vi "ErrorLog_GetErrors.vi"(7 "Owner":string, 8 "error in (no error)":errorcluster, 11 "reference in":refnum<class "ErrorLog.lvclass">) -> (0 "error out":errorcluster, 1 "Errors since last call":string, 2 "New Errors":bool, 3 "reference out":refnum<class "ErrorLog.lvclass">, 4 "Errors since last clear":string, 5 "Uncleared Errors":bool)   [LabVIEW 2014, in "ErrorLog.lvclass"]
uses:
  ErrorLog.lvclass
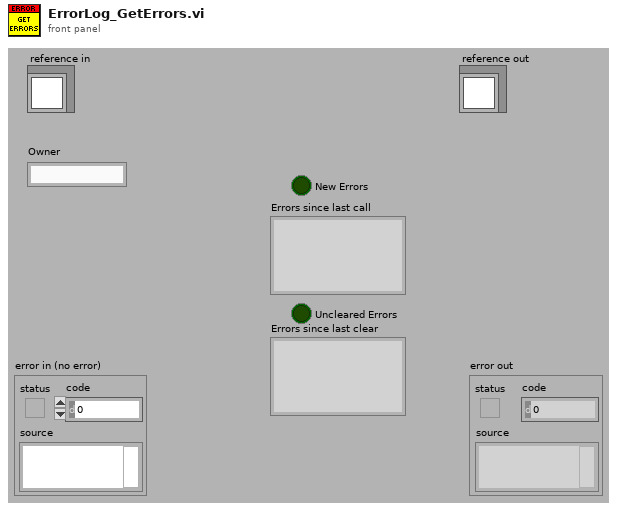
[diagram p1: front panel]
types:
  T1 = typedef "ErrorLog.lvclass/ObjectAttributes.ctl" = cluster{"ErrorFile":path, "Supress Consecutive Duplicates":bool, "Errors":string, "Quit":bool, "Errors since last call":string, "Last Recorded Error":string, "ErrorPath":path, "PossiblePaths":path[], "BaseFileName":string, "Max Log Files":i32, "ErrorFile Index":i32, "Max File Size":i64}
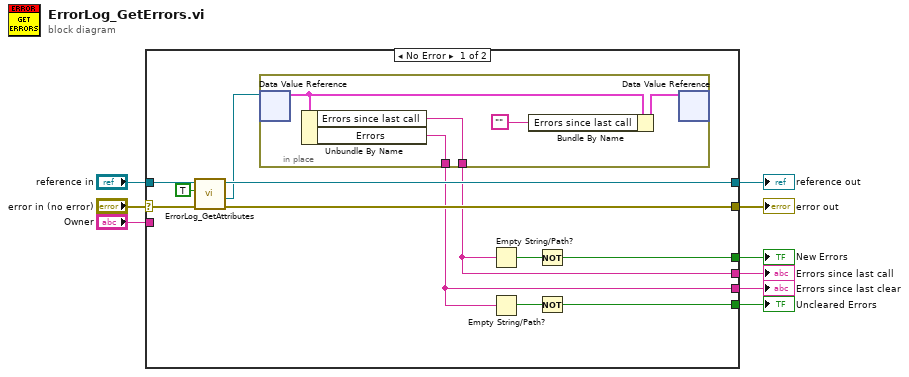
[diagram p0: block diagram]
diagram:
  n1 = case shown="No Error" "error in (no error)" {
    selector: "error in (no error)" -> [w21 w28]
    tunnel: [w19 w28] -> w8
    tunnel: [w14 w27] -> w6
    tunnel: "reference in" -> [w20 w27]
    tunnel: [w11 _] -> w5
    tunnel: [w10 _] -> w4
    tunnel: "Owner" -> [_ _]
    tunnel: [w16 _] -> w2
    tunnel: [w15 _] -> w1
    frame No Error {
      n2 = call "ErrorLog_GetAttributes.vi"("error in (no error)"=w21, "OnlyGetDvrReference(False)"=TRUE, "reference in"=w20) -> ("error out"=w19:errorcluster, "DataRef"=w12:refnum<data-value>, "reference out"=w14:refnum<class "ErrorLog.lvclass">)  [unwired: 5 in, 1 out]
      n3 = in-place {
        in-place-border: [w26] -> w11
        in-place-border: [w25] -> w10
        n4 = in-place-dvr #1(w12) -> (w24:T1)  [unwired: 1 out]
        n5 = Unbundle By Name(w24) -> ("Errors since last call"=w26:string, "Errors"=w25:string)
        n6 = Bundle By Name(cluster=w24, "Errors since last call"="") -> (w23:T1)
        n7 = in-place-dvr #1(w23) -> ()  [unwired: 2 out]
      }
      n8 = Empty String/Path?(string/path=w11) -> (empty?=w18:bool)
      n9 = Empty String/Path?(string/path=w10) -> (empty?=w17:bool)
      n10 = Not(x=w18) -> (.not. x?=w15:bool)
      n11 = Not(x=w17) -> (.not. x?=w16:bool)
    }
    frame Error {
    }
  }
  "error out" <- w8
  "reference out" <- w6
  "Errors since last call" <- w5
  "New Errors" <- w1
  "Errors since last clear" <- w4
  "Uncleared Errors" <- w2
